vi "Elevator_Controller.vi"(8 "error in (no error)":errorcluster) -> (0 "error out":errorcluster)   [LabVIEW 2013]
doc: "Controller for the application. Sends and receives messages from the modules."
uses:
  Display Console/Display_Data.ctl
  User Console/Requests.ctl
  Sensor Interface/Sensor_Station.ctl
  controller_Data.ctl
  Controller_Enum.ctl
  Messaging/Msg_Control.ctl
  User Console/User_Console_enum.ctl
  Display Console/Display_Enum.ctl
  Database/DB_control.ctl
  Database/DB_Data.ctl
  Sensor Interface/Sensor_Enum.ctl
  Hardware_Enum.ctl
panel:
  in  "Controller_Enum":T1
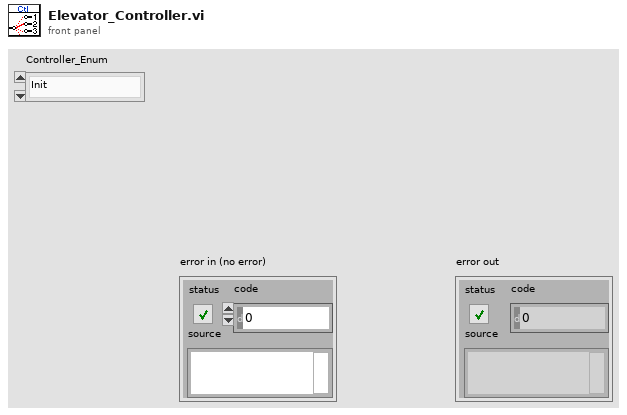
[diagram p1: front panel]
types:
  T1 = typedef "Controller_Enum.ctl" = enum16{"Init", "Wait_Start", "Start_State", "Moving", "Wait_Sensor_move", "Analysis", "Continue_Move", "Stop_Floor", "Doors", "Doors_Shut", "No Requests", "Emergency", "Terminate"}
  T2 = typedef "Msg_Control.ctl" = enum16{"Init_Msg", "Sent_Inits", "Get_Ref", "Close_Ref"}
  T3 = typedef "DB_control.ctl" = enum16{"Initi_FGV", "Open", "Get_Data", "Write_Data", "Write_File", "Close_File"}
  T4 = typedef "controller_Data.ctl" = cluster{"Requests":T5, "Display_Data":T6, "Slide":T7, "DB Data":T8}
  T5 = typedef "Requests.ctl" = cluster{"1 u":bool, "3 u":bool, "2 u":bool, "2 d":bool, "4 d":bool, "3 d":bool, "1":bool, "2":bool, "3":bool, "4":bool}
  T6 = typedef "Display_Data.ctl" = cluster{"Timing":dbl, "Current Floor":u8, "Up":bool, "Down":bool, "Door Open":bool, "Emergency":bool}
  T7 = typedef "Sensor_Station.ctl" = u8
  T8 = typedef "DB_Data.ctl" = cluster{"Door Open Time":dbl, "Travel Time":dbl, "Inactivity Time":dbl, "Door Close Time ":dbl, "Hardware Bit Sensor":T9, "Hardware Bit User console":T9, "Hardware Bit Display":T9, "Controller Bit Display":T9}
  T9 = typedef "Hardware_Enum.ctl" = enum16{"Simulation", "Hardware"}
  T10 = cluster{"queue out":refnum<queue>, "queue out":refnum<queue>, "queue out":refnum<queue>}
  T11 = typedef "Display_Enum.ctl" = enum16{"Init", "Update1", "Update2(etc)", "Teminate"}
  T12 = typedef "User_Console_enum.ctl" = enum16{"Init", "Idle", "Send_Request", "Send_Door", "Send_Emergency", "Receive_Request", "Receive_Door", "Receive_Emergency", "Terminate"}
  T13 = typedef "Sensor_Enum.ctl" = enum16{"Init", "Idle", "Send_Position", "Terminate"}
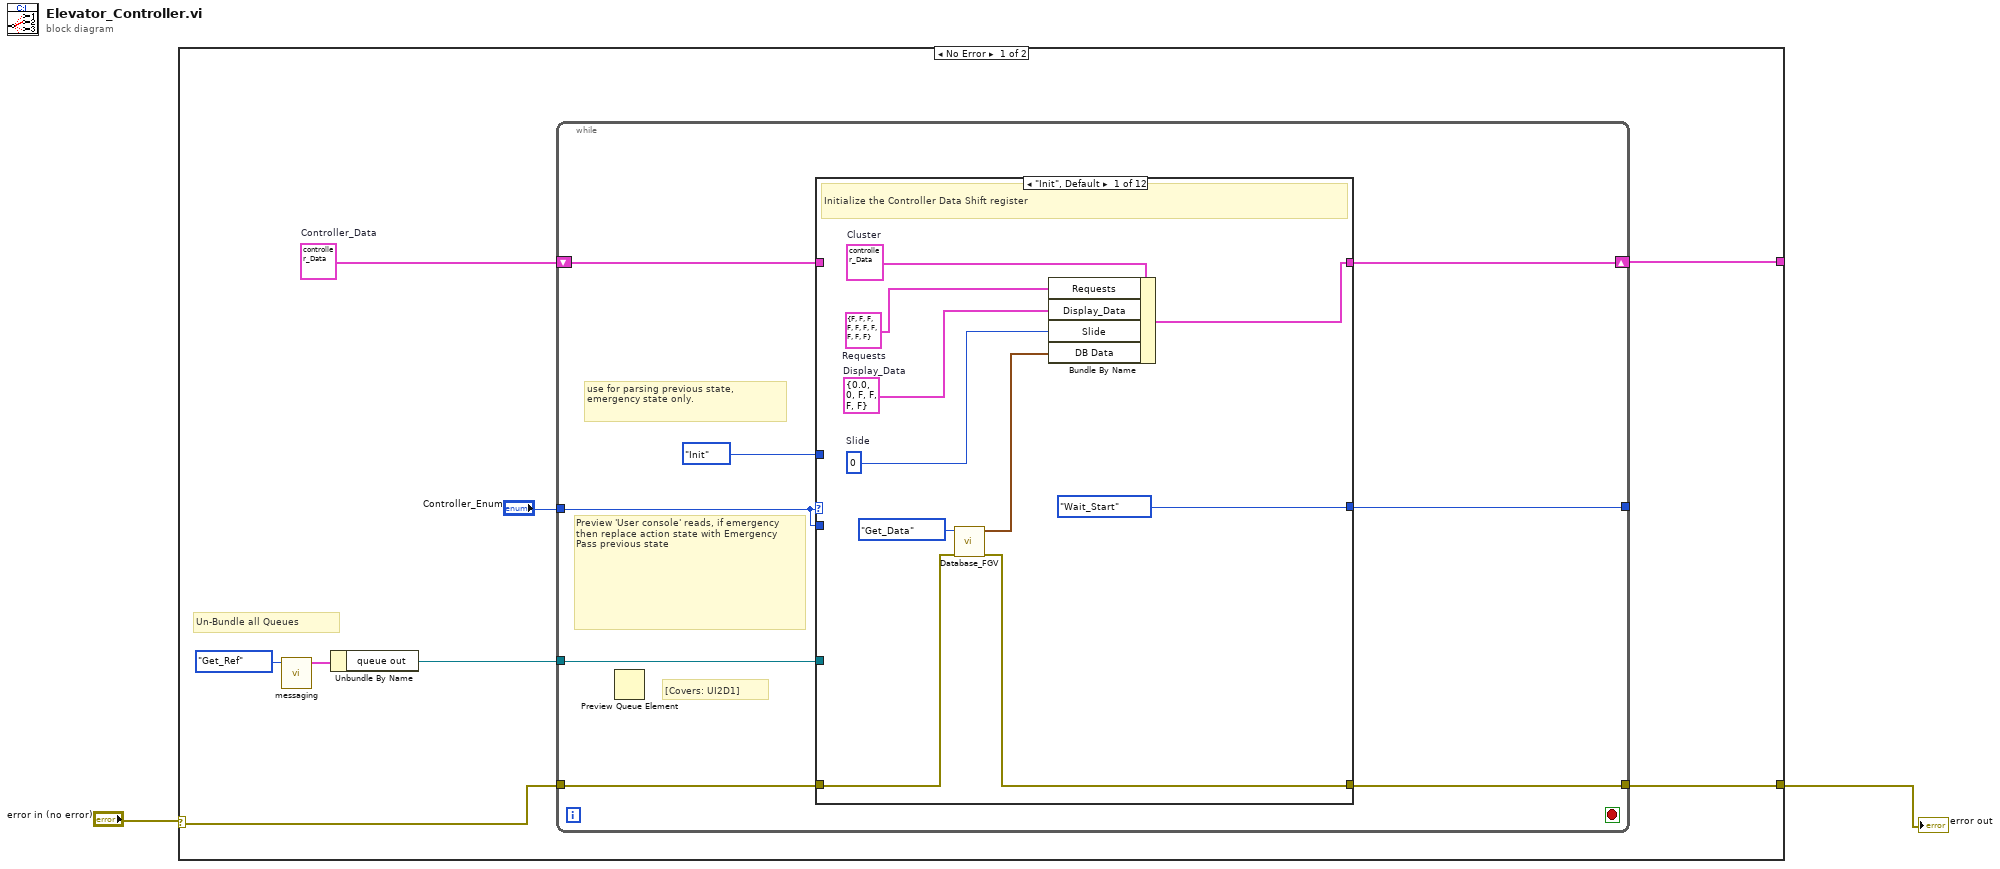
[diagram p0: block diagram]
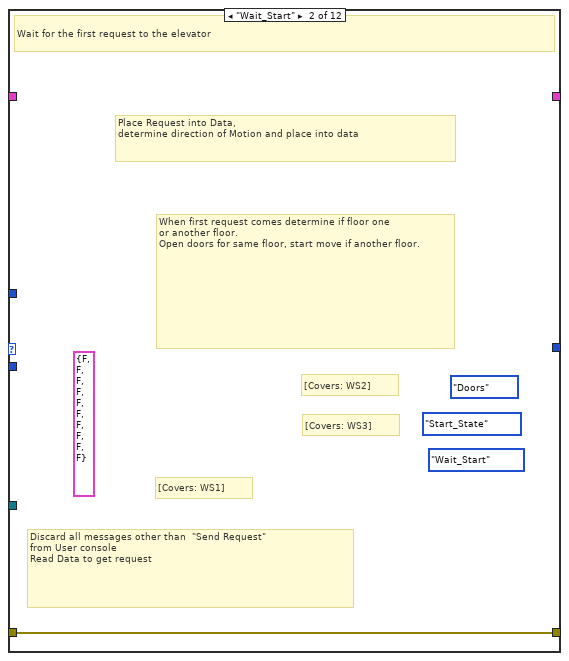
[diagram p2: hidden frame]
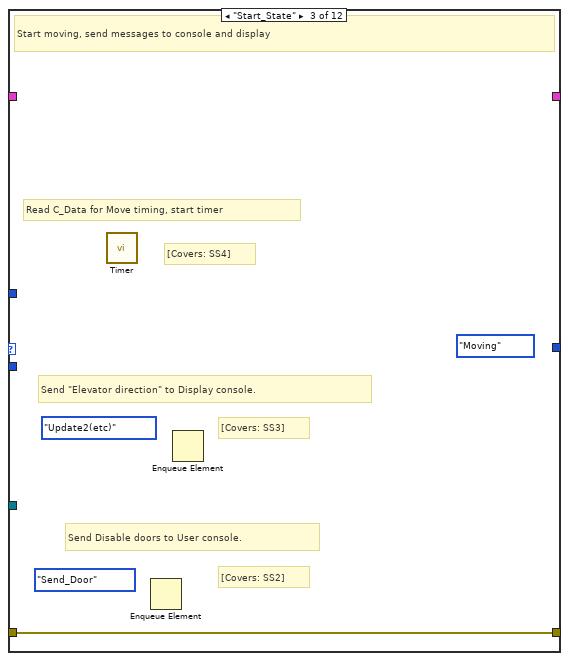
[diagram p3: hidden frame]
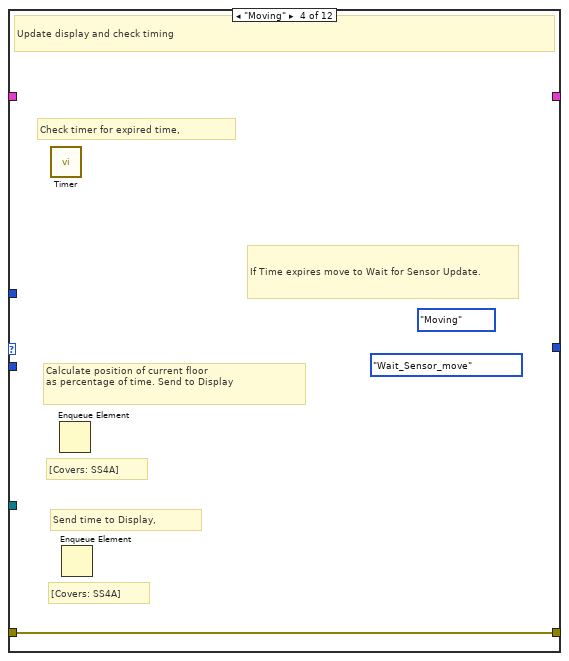
[diagram p4: hidden frame]
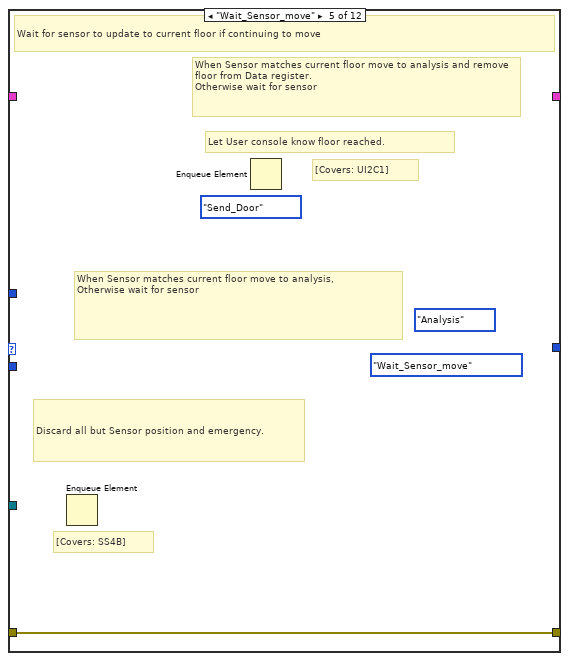
[diagram p5: hidden frame]
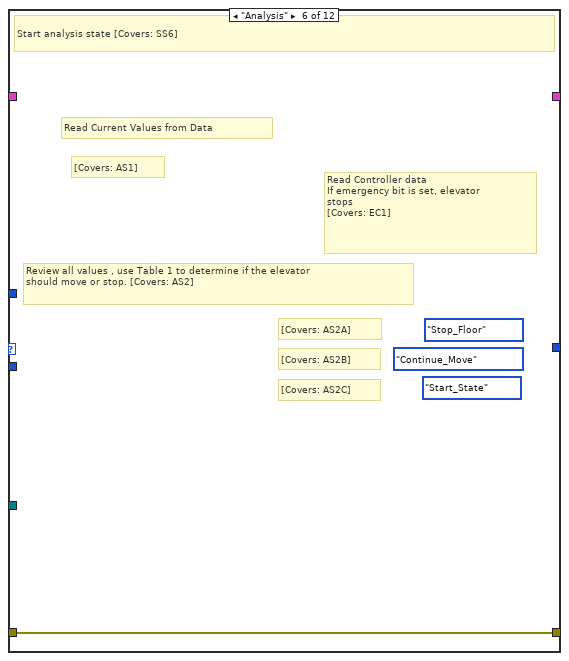
[diagram p6: hidden frame]
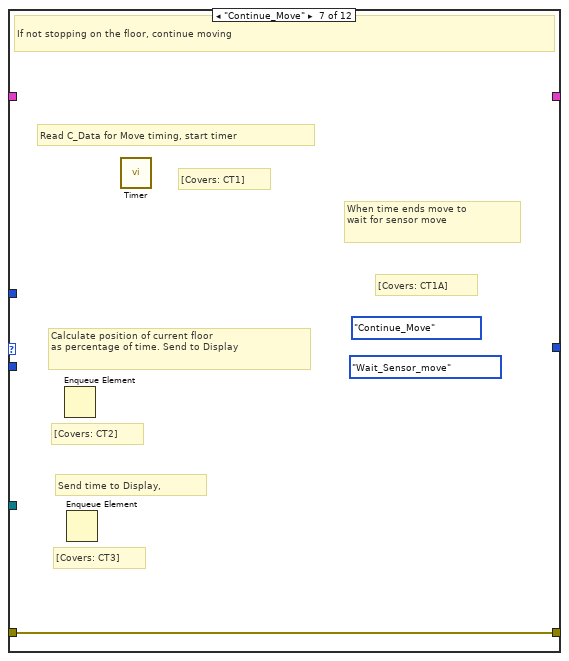
[diagram p7: hidden frame]
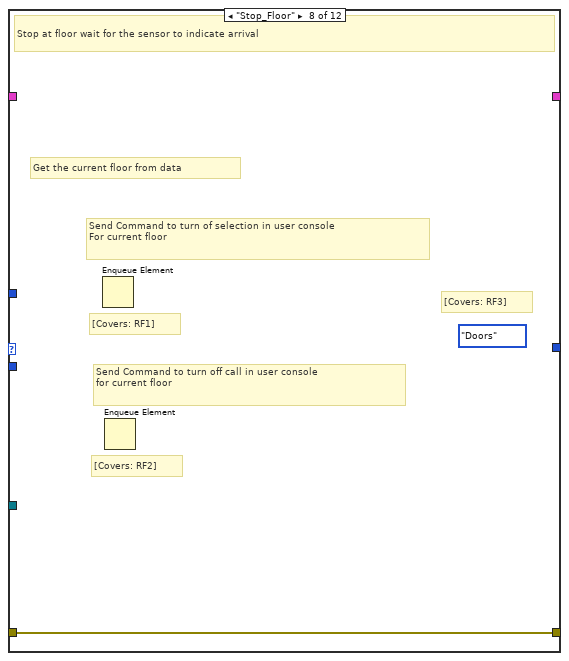
[diagram p8: hidden frame]
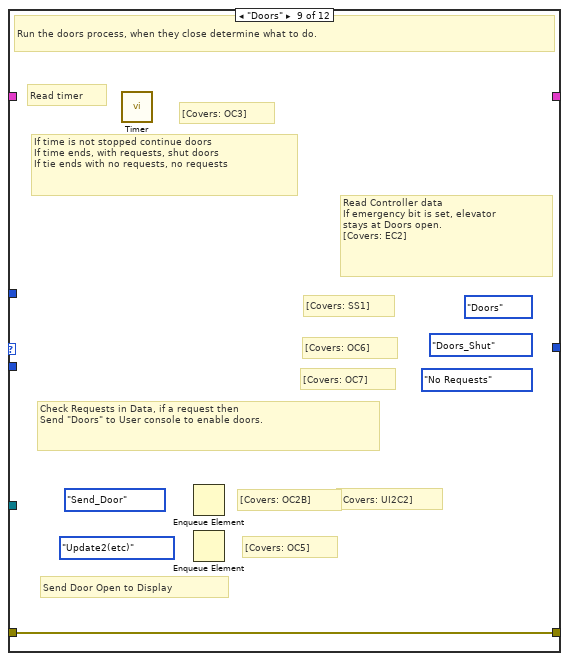
[diagram p9: hidden frame]
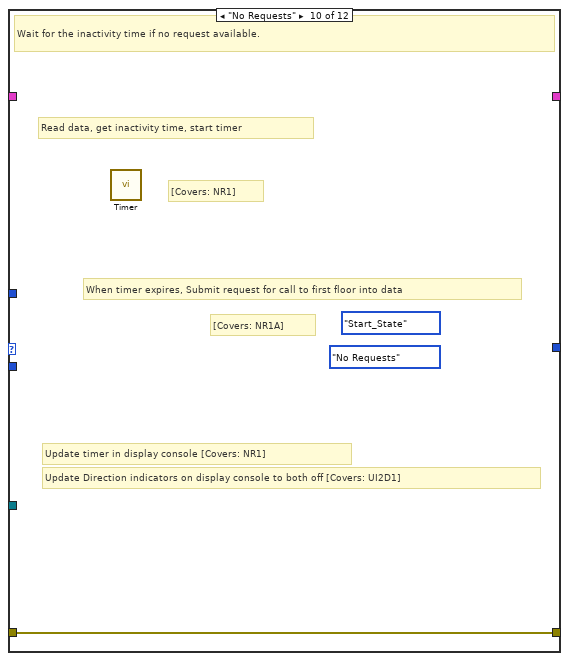
[diagram p10: hidden frame]
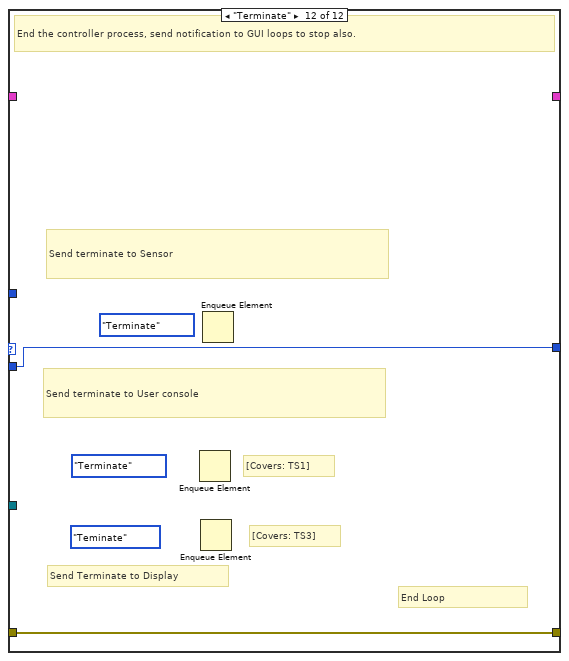
[diagram p12: hidden frame]
diagram:
  n1 = case shown="No Error" "error in (no error)" {
    selector: "error in (no error)" -> [w9 w41]
    tunnel: [w8 w41] -> w1
    tunnel: [w7 _] -> _
    frame No Error {
      w6 = T4 {"Requests"={"1 u"=FALSE, "3 u"=FALSE, "2 u"=FALSE, "2 d"=FALSE, "4 d"=FALSE, "3 d"=FALSE, "1"=FALSE, "2"=FALSE, "3"=FALSE, "4"=FALSE}, "Display_Data"={"Timing"=0.0, "Current Floor"=0, "Up"=FALSE, "Down"=FALSE, "Door Open"=FALSE, "Emergency"=FALSE}, "Slide"=0, "DB Data"={"Door Open Time"=0.0, "Travel Time"=0.0, "Inactivity Time"=0.0, "Door Close Time "=0.0, "Hardware Bit Sensor"=enum."Simulation", "Hardware Bit User console"=enum."Simulation", "Hardware Bit Display"=enum."Simulation", "Controller Bit Display"=enum."Simulation"}}  # Controller_Data
      # "Un-Bundle all Queues"
      n2 = call "messaging.vi"("Message_Control"=Msg_Control."Get_Ref") -> ("REfs Out"=w4:T10)  [unwired: 9 in, 1 out]
      n3 = Unbundle By Name(w4) -> ("queue out"=w3:refnum<queue>)
      n4 = while {
        tunnel: "Controller_Enum" -> [w14]
        tunnel: w9 -> [w18]
        tunnel: [w17] -> w8
        shift-right: [w16] -> w7
        shift-left: w6 -> [w15]
        tunnel: [w13] -> _
        tunnel: w3 -> [w12]
        stop <- _ stop-if-true
        # "[Covers: UI2D1]"
        # "use for parsing previous state, \nemergency state only."
        # "Preview 'User console' reads, if emergency\nthen replace action state with Emergency\nPass previous state"
        n5 = Preview Queue Element() -> ()  [unwired: 3 in, 4 out]
        n6 = case shown="\"Init\", Default" w14 {
          tunnel: w18 -> [w20 w29 w30 w31 w32 w33 w34 w35 w36 w37 w38 w40]
          tunnel: [w19 w29 w30 w31 w32 w33 w34 w35 w36 w37 w38 w40] -> w17
          tunnel: [w24 _ _ _ _ _ _ _ _ _ _ _] -> w16
          tunnel: w15 -> [_ _ _ _ _ _ _ _ _ _ _ _]
          tunnel: w14 -> [_ _ _ _ _ _ _ _ _ _ _ w39]
          tunnel: [Controller_Enum."Wait_Start" ("Controller_Enum 2") _ _ _ _ _ _ _ _ _ _ w39] -> w13
          tunnel: w12 -> [_ _ _ _ _ _ _ _ _ _ _ _]
          tunnel: Controller_Enum."Init" ("Controller_Enum 2") -> [_ _ _ _ _ _ _ _ _ _ _ _]
          frame "Init", Default {
            w28 = T4 {"Requests"={"1 u"=FALSE, "3 u"=FALSE, "2 u"=FALSE, "2 d"=FALSE, "4 d"=FALSE, "3 d"=FALSE, "1"=FALSE, "2"=FALSE, "3"=FALSE, "4"=FALSE}, "Display_Data"={"Timing"=0.0, "Current Floor"=0, "Up"=FALSE, "Down"=FALSE, "Door Open"=FALSE, "Emergency"=FALSE}, "Slide"=0, "DB Data"={"Door Open Time"=0.0, "Travel Time"=0.0, "Inactivity Time"=0.0, "Door Close Time "=0.0, "Hardware Bit Sensor"=enum."Simulation", "Hardware Bit User console"=enum."Simulation", "Hardware Bit Display"=enum."Simulation", "Controller Bit Display"=enum."Simulation"}}  # Cluster
            w25 = T7 0  # Slide
            w27 = T5 {"1 u"=FALSE, "3 u"=FALSE, "2 u"=FALSE, "2 d"=FALSE, "4 d"=FALSE, "3 d"=FALSE, "1"=FALSE, "2"=FALSE, "3"=FALSE, "4"=FALSE}  # Requests
            w26 = T6 {"Timing"=0.0, "Current Floor"=0, "Up"=FALSE, "Down"=FALSE, "Door Open"=FALSE, "Emergency"=FALSE}  # Display_Data
            # "Initialize the Controller Data Shift register"
            n7 = call "Database_FGV.vi"("error in (no error)"=w20, "DB Control"=DB_control."Get_Data") -> ("error out"=w19:errorcluster, "DB Data Out"=w21:T8)  [unwired: 8 in]
            n8 = Bundle By Name(cluster=w28, "Requests"=w27, "Display_Data"=w26, "Slide"=w25, "DB Data"=w21) -> (w24:T4)
          }
          frame "Wait_Start" {
            (unwired) T5 {"1 u"=FALSE, "3 u"=FALSE, "2 u"=FALSE, "2 d"=FALSE, "4 d"=FALSE, "3 d"=FALSE, "1"=FALSE, "2"=FALSE, "3"=FALSE, "4"=FALSE} ("Requests")
            (unwired) Controller_Enum."Doors" ("Controller_Enum 2")
            (unwired) Controller_Enum."Wait_Start" ("Controller_Enum 2")
            (unwired) Controller_Enum."Start_State" ("Controller_Enum 2")
            # "Place Request into Data, \ndetermine direction of Motion and place into data"
            # "[Covers: WS3]"
            # "[Covers: WS2]"
            # "[Covers: WS1]"
            # "When first request comes determine if floor one\nor another floor.\nOpen doors for same floor, start move if another floor."
            # "Discard all messages other than  \"Send Request\"\nfrom User console\nRead Data to get request"
            # "Wait for the first request to the elevator"
          }
          frame "Start_State" {
            (unwired) Controller_Enum."Moving" ("Controller_Enum 2")
            (unwired) Display_Enum."Update2(etc)" ("Display_Enum")
            (unwired) User_Console_enum."Send_Door" ("User_console_Enum")
            # "[Covers: SS4]"
            # "Read C_Data for Move timing, start timer"
            # "[Covers: SS3]"
            # "Send \"Elevator direction\" to Display console."
            # "[Covers: SS2]"
            # "Send Disable doors to User console."
            # "Start moving, send messages to console and display"
            n9 = call "Timer.vi"() -> ()  [unwired: 10 in, 2 out]
            n10 = Enqueue Element() -> ()  [unwired: 4 in, 3 out]
            n11 = Enqueue Element() -> ()  [unwired: 4 in, 3 out]
          }
          frame "Moving" {
            (unwired) Controller_Enum."Wait_Sensor_move" ("Controller_Enum 2")
            (unwired) Controller_Enum."Moving" ("Controller_Enum 2")
            # "[Covers: SS4A]"
            # "Calculate position of current floor\nas percentage of time. Send to Display"
            # "If Time expires move to Wait for Sensor Update."
            # "[Covers: SS4A]"
            # "Send time to Display,"
            # "Check timer for expired time,"
            # "Update display and check timing"
            n12 = call "Timer.vi"() -> ()  [unwired: 10 in, 2 out]
            n13 = Enqueue Element() -> ()  [unwired: 4 in, 3 out]
            n14 = Enqueue Element() -> ()  [unwired: 4 in, 3 out]
          }
          frame "Wait_Sensor_move" {
            (unwired) User_Console_enum."Send_Door" ("User_console_Enum")
            (unwired) Controller_Enum."Wait_Sensor_move" ("Controller_Enum 2")
            (unwired) Controller_Enum."Analysis" ("Controller_Enum 2")
            # "[Covers: UI2C1]"
            # "Let User console know floor reached."
            # "When Sensor matches current floor move to analysis and remove floor from Data register.\nOtherwise wait for sensor"
            # "When Sensor matches current floor move to analysis,\nOtherwise wait for sensor"
            # "[Covers: SS4B]"
            # "Discard all but Sensor position and emergency."
            # "Wait for sensor to update to current floor if continuing to move"
            n15 = Enqueue Element() -> ()  [unwired: 4 in, 3 out]
            n16 = Enqueue Element() -> ()  [unwired: 4 in, 3 out]
          }
          frame "Analysis" {
            (unwired) Controller_Enum."Start_State" ("Controller_Enum")
            (unwired) Controller_Enum."Continue_Move" ("Controller_Enum")
            (unwired) Controller_Enum."Stop_Floor" ("Controller_Enum")
            # "Read Controller data \nIf emergency bit is set, elevator\nstops \n[Covers: EC1]"
            # "[Covers: AS2C]"
            # "[Covers: AS2B]"
            # "[Covers: AS2A]"
            # "Review all values , use Table 1 to determine if the elevator\nshould move or stop. [Covers: AS2]"
            # "[Covers: AS1]"
            # "Read Current Values from Data"
            # "Start analysis state [Covers: SS6]"
          }
          frame "Continue_Move" {
            (unwired) Controller_Enum."Wait_Sensor_move" ("Controller_Enum 2")
            (unwired) Controller_Enum."Continue_Move" ("Controller_Enum 2")
            # "When time ends move to \nwait for sensor move"
            # "[Covers: CT2]"
            # "Calculate position of current floor\nas percentage of time. Send to Display"
            # "[Covers: CT3]"
            # "Send time to Display,"
            # "[Covers: CT1A]"
            # "[Covers: CT1]"
            # "Read C_Data for Move timing, start timer"
            # "If not stopping on the floor, continue moving"
            n17 = Enqueue Element() -> ()  [unwired: 4 in, 3 out]
            n18 = Enqueue Element() -> ()  [unwired: 4 in, 3 out]
            n19 = call "Timer.vi"() -> ()  [unwired: 10 in, 2 out]
          }
          frame "Stop_Floor" {
            (unwired) Controller_Enum."Doors" ("Controller_Enum 2")
            # "[Covers: RF3]"
            # "[Covers: RF1]"
            # "Send Command to turn of selection in user console\nFor current floor"
            # "[Covers: RF2]"
            # "Send Command to turn off call in user console\nfor current floor"
            # "Get the current floor from data"
            # "Stop at floor wait for the sensor to indicate arrival"
            n20 = Enqueue Element() -> ()  [unwired: 4 in, 3 out]
            n21 = Enqueue Element() -> ()  [unwired: 4 in, 3 out]
          }
          frame "Doors" {
            (unwired) User_Console_enum."Send_Door" ("User_console_Enum")
            (unwired) Display_Enum."Update2(etc)" ("Display_Enum")
            (unwired) Controller_Enum."No Requests" ("Controller_Enum 2")
            (unwired) Controller_Enum."Doors_Shut" ("Controller_Enum 2")
            (unwired) Controller_Enum."Doors" ("Controller_Enum 2")
            # "[Covers: UI2C2]"
            # "[Covers: SS1]"
            # "Read Controller data \nIf emergency bit is set, elevator\nstays at Doors open. \n[Covers: EC2]"
            # "Send Door Open to Display"
            # "[Covers: OC5]"
            # "[Covers: OC6]"
            # "[Covers: OC7]"
            # "If time is not stopped continue doors\nIf time ends, with requests, shut doors\nIf tie ends with no requests, no requests"
            # "[Covers: OC3]"
            # "Read timer"
            # "[Covers: OC2B]"
            # "Check Requests in Data, if a request then  \nSend \"Doors\" to User console to enable doors."
            # "Run the doors process, when they close determine what to do."
            n22 = call "Timer.vi"() -> ()  [unwired: 10 in, 2 out]
            n23 = Enqueue Element() -> ()  [unwired: 4 in, 3 out]
            n24 = Enqueue Element() -> ()  [unwired: 4 in, 3 out]
          }
          frame "No Requests" {
            (unwired) Controller_Enum."No Requests" ("Controller_Enum 2")
            (unwired) Controller_Enum."Start_State" ("Controller_Enum 2")
            # "Update Direction indicators on display console to both off [Covers: UI2D1]"
            # "[Covers: NR1A]"
            # "When timer expires, Submit request for call to first floor into data"
            # "Update timer in display console [Covers: NR1]"
            # "[Covers: NR1]"
            # "Read data, get inactivity time, start timer"
            # "Wait for the inactivity time if no request available."
            n25 = call "Timer.vi"() -> ()  [unwired: 10 in, 2 out]
          }
          frame "Emergency" {
            # "If turning Emergency off, \nPlace Initialize into shift register\n[Covers: EC3]"
            # "Set Emergency Bit to new value\nPlace previous state back in shift register"
            # "Set emergency bits, continue with process (move to stop or remain stopped)"
          }
          frame "Terminate" {
            (unwired) Sensor_Enum."Terminate" ("Sensor_Enum")
            (unwired) Display_Enum."Teminate" ("Display_Enum")
            (unwired) User_Console_enum."Terminate" ("User_console_Enum")
            # "Send terminate to Sensor"
            # "End Loop"
            # "Send Terminate to Display"
            # "[Covers: TS3]"
            # "[Covers: TS1]"
            # "Send terminate to User console"
            # "End the controller process, send notification to GUI loops to stop also."
            n26 = Enqueue Element() -> ()  [unwired: 4 in, 3 out]
            n27 = Enqueue Element() -> ()  [unwired: 4 in, 3 out]
            n28 = Enqueue Element() -> ()  [unwired: 4 in, 3 out]
          }
        }
      }
    }
    frame Error {
    }
  }
  "error out" <- w1
